vi "ROI entry-Event handler-Whole plane.vi"   [LabVIEW 2013]
uses:
  ROI Entry screen/Globals/gl_ROI Entry UI globals.vi
types:
  T1 = typedef "ROI entry screen ctrl refs cluster.ctl" = cluster{"Done button":refnum<vi>, "Imaging button":refnum<vi>, "Acquisition button":refnum<vi>, "POI dwell time (us)":refnum<vi>, "Scan dwell time per pixel (us)":refnum<vi>, "# of planes":refnum<vi>, "Zoom":refnum<vi>, "Equal size":refnum<vi>, "Channel":refnum<vi>, "Image Display":refnum<vi>, "Z-Plane Selector":refnum<vi>, "Number of lines left":refnum<vi>, "Z-stack folder path":refnum<vi>, "POI Density":refnum<vi>, "Arb Plane Entry":refnum<vi>, "Whole plane":refnum<vi>, "Clear Last":refnum<vi>, "Clear All":refnum<vi>, "Trial Length (sec)":refnum<vi>, "Palette Type":refnum<vi>, "Intensity slider":refnum<vi>, "# POI":refnum<vi>, "Max Z Proj":refnum<vi>, "Zplane ind":refnum<vi>, "Wavelength (nm)":refnum<vi>, "Number of Trials":refnum<vi>, "Funct stim.trig.enable":refnum<vi>, "Funct stim.trig.delay (s)":refnum<vi>, "Line Mode":refnum<vi>, "Step size (µm)":refnum<vi>, "ROI move mode":refnum<vi>, "Cool-down time (s)":refnum<vi>, "Enable cool-down time":refnum<vi>, "Motor Z ind. (um)":refnum<vi>, "AOL Z ind. (um)":refnum<vi>}
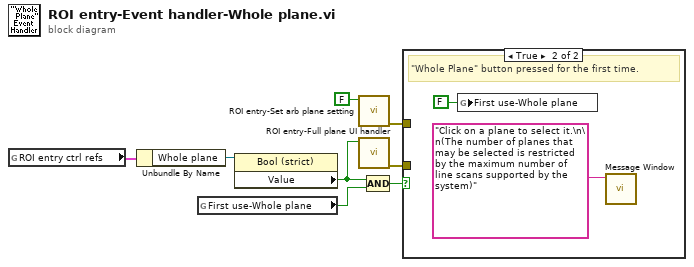
[diagram p0: block diagram]
diagram:
  n1 = global read "gl_ROI Entry UI globals.vi" "ROI entry ctrl refs"() -> (w3:T1)
  n2 = Unbundle By Name(w3) -> ("Whole plane"=w4:refnum<vi>)
  n3 = global read "gl_ROI Entry UI globals.vi" "First use-Whole plane"() -> (w6:bool)
  n4 = property on="Property Node" class="Bool (strict)"(reference=w4) -> ("Value"=w2:bool)  [unwired: 1 in, 2 out]
  n5 = call "ROI entry-Set arb plane setting.vi"("\"Arb plane entry\" button's value"=FALSE ("\"Arb plane entry\" button's value")) -> ("error out"=w8:errorcluster)  [unwired: 10 in]
  n6 = call "ROI entry-Full plane UI handler.vi"("Whole plane mode ON"=w2) -> ("error out"=w1:errorcluster)  [unwired: 10 in]
  n7 = Compound Arithmetic op=AND(w2, w6) -> (w5:bool)
  n8 = case shown="True" w5 {
    tunnel: w8 -> [_ _]
    tunnel: w1 -> [_ _]
    frame False {
    }
    frame True {
      # "\"Whole Plane\" button pressed for the first time."
      n9 = global write "gl_ROI Entry UI globals.vi" "First use-Whole plane"(FALSE ("First call")) -> ()
      n10 = call "Message Window.vi"("Message string"="Click on a plane to select it.\n\n(The number of planes that may be selected is restricted by the maximum number of line scans supported by the system)") -> ()  [unwired: 10 in, 1 out]
    }
  }
